vi "Process Move.vi"(9 "Direction":T1, 10 "Action":T2, 11 "Base Builder In":refnum<class "Base Builder.lvclass">) -> (2 "Replicated":refnum<class "Base Builder.lvclass">, 3 "Base Builder Out":refnum<class "Base Builder.lvclass">)   [LabVIEW 2015, in "Base Builder.lvclass"]
uses:
  Base Builder/Base Builder.lvclass
  Type Defs/Action Enum.ctl
  Type Defs/Direction Enum.ctl
  Base Builder/Base Builder.lvclass/Base Builder.ctl
  Square/Board Size.vi
  SubVIs/Read-Only Globals.vi
  Common/Common.lvlib
  Type Defs/SB Type Defs.lvlib
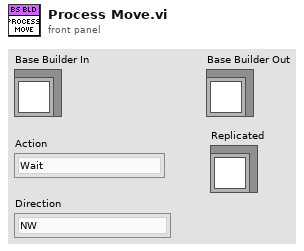
[diagram p1: front panel]
types:
  T1 = typedef "SB Type Defs.lvlib/Direction Enum.ctl" = enum16{"NW", "N", "NE", "E", "SE", "S", "SW", "W"}
  T2 = typedef "SB Type Defs.lvlib/Action Enum.ctl" = enum16{"Wait", "Move", "Attack", "Replicate"}
  T3 = typedef "Common.lvlib/Position.ctl" = cluster{"Column":i32, "Row":i32}
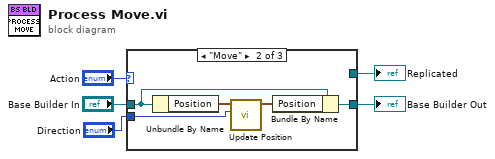
[diagram p0: block diagram]
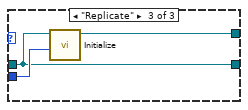
[diagram p3: hidden frame]
diagram:
  n1 = case shown="\"Move\"" "Action" {
    tunnel: "Base Builder In" -> [w6 w8 w12]
    tunnel: [w6 w9 w12] -> w3
    tunnel: "Direction" -> [_ w11 w14]
    tunnel: [_ _ w13] -> w1
    frame Default {
    }
    frame "Move" {
      n2 = Unbundle By Name(w8) -> ("Position"=w10:cluster{"Column":i32, "Row":i32})
      n3 = call "Update Position.vi"("Direction"=w11, "Position in"=w10) -> ("Position out"=w7:T3)  [unwired: 9 in]
      n4 = Bundle By Name(cluster=w8, "Position"=w7) -> (w9:refnum<class "Base Builder.lvclass">)
    }
    frame "Replicate" {
      n5 = call-dynamic "Initialize.vi"("Spawn Direction"=w14, "Base Builder in"=w12) -> ("Base Builder out"=w13:refnum<class "Base Builder.lvclass">)  [unwired: 8 in, 1 out]
    }
  }
  "Base Builder Out" <- w3
  "Replicated" <- w1
